vi "Translator.vi"(0 "Input":variant, 11 "error in (no error)":errorcluster) -> (4 "Output":variant, 15 "error out":errorcluster)   [LabVIEW 2014, in "Arduino LiquidCrystal Wrapper.lvlib"]
doc: "An example of how to create the Translator to convert the LabVIEW VIs to Arduino C code."
uses:
  <vilib>/Aledyne-TSXperts/Arduino Compatible Compiler for LabVIEW/addons/Arduino LiquidCrystal Wrapper/Arduino LiquidCrystal Wrapper.lvlib
panel:
  out "Outputs":string[](array[string])
  out "Inputs":string[](array[string])
  out "Output Datatypes":string[](array[string])
  out "Input Datatypes":string[](array[string])
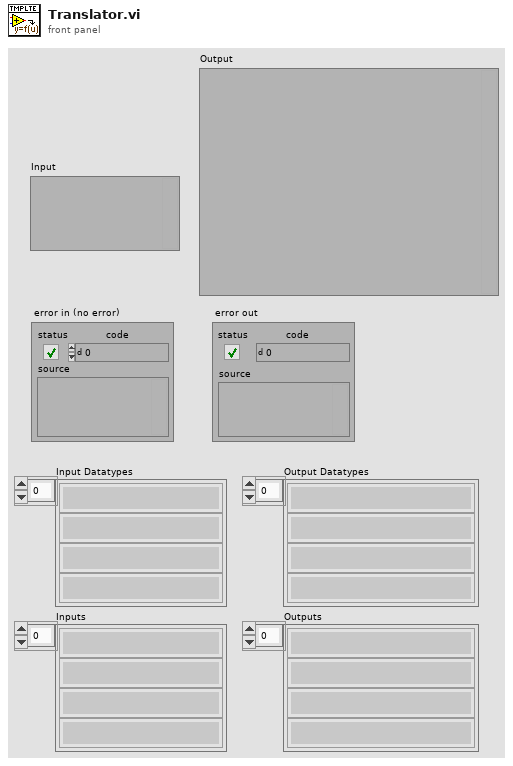
[diagram p1: front panel]
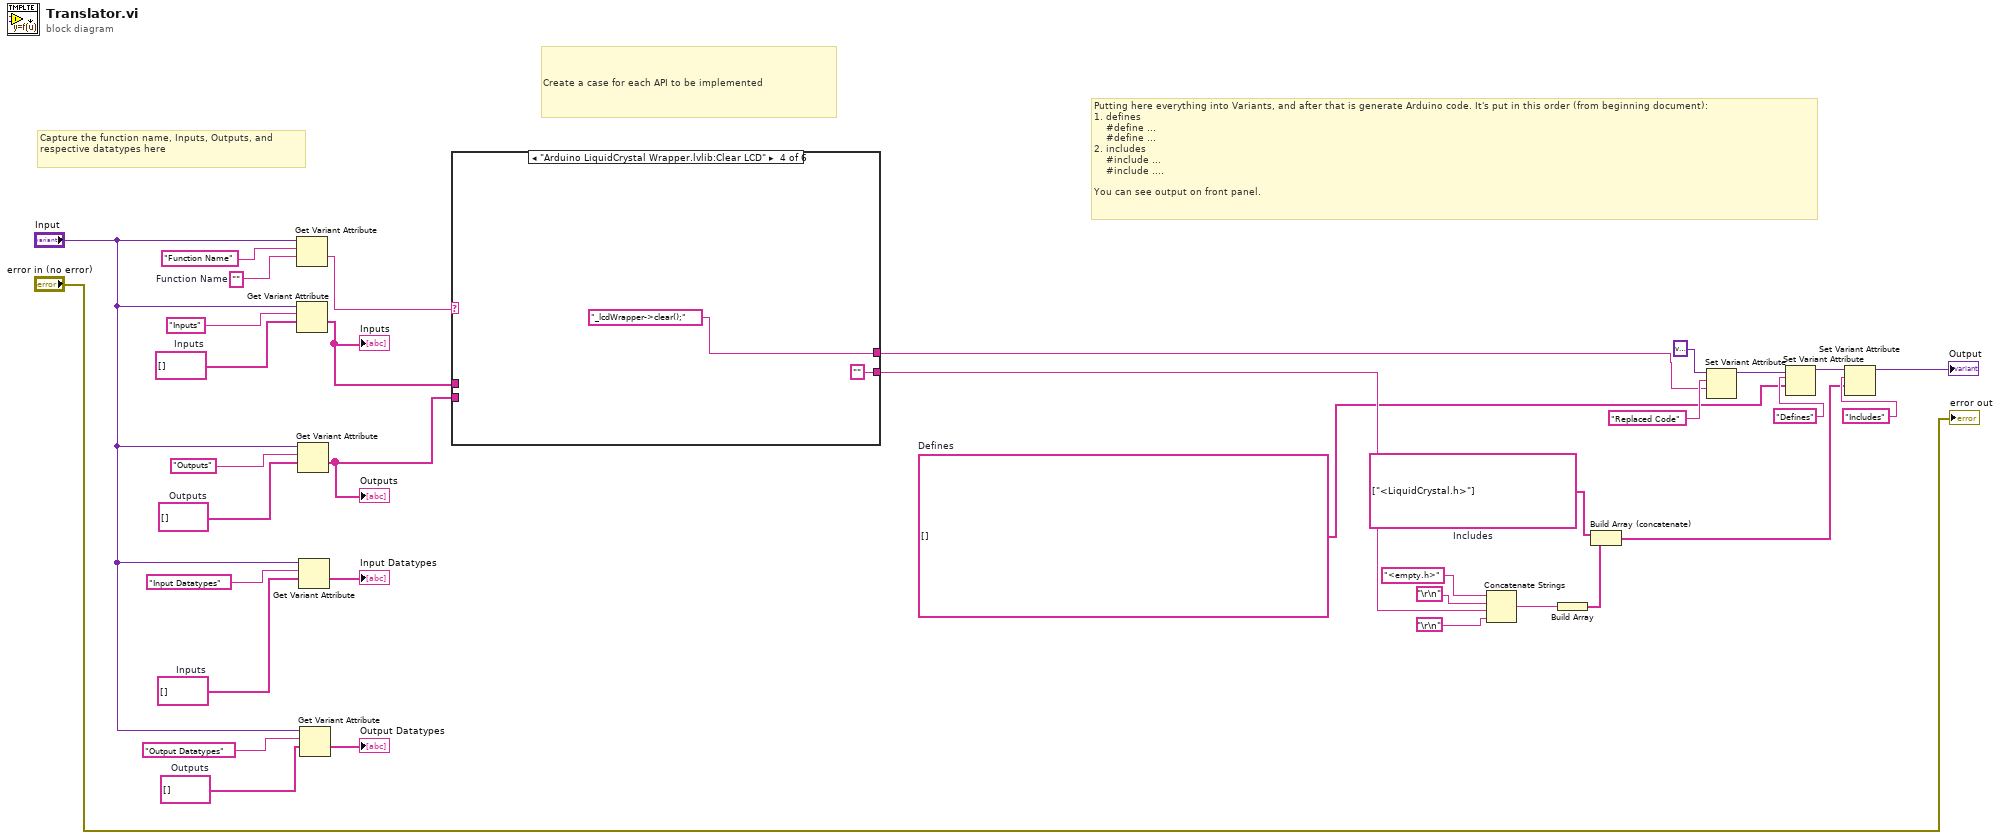
[diagram p0: block diagram]
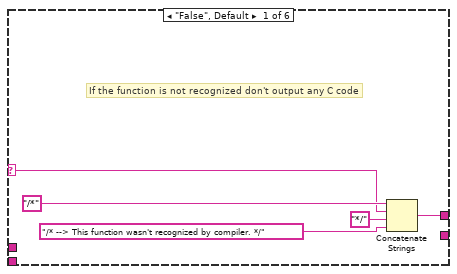
[diagram p2: hidden frame]
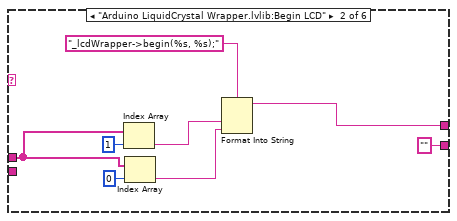
[diagram p3: hidden frame]
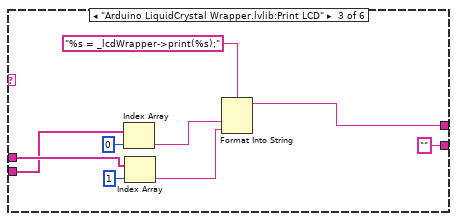
[diagram p4: hidden frame]
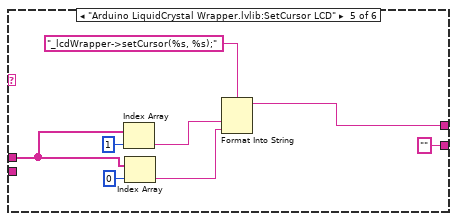
[diagram p5: hidden frame]
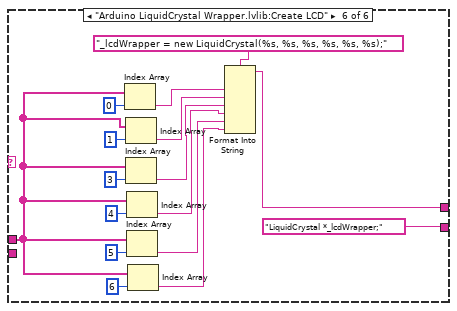
[diagram p6: hidden frame]
diagram:
  w1 = string[] []  # Defines
  w21 = string[] []  # Outputs
  w22 = string[] []  # Inputs
  w3 = string[] ["<LiquidCrystal.h>"]  # Includes
  w30 = string[] []  # Outputs
  w31 = string[] []  # Inputs
  w32 = ""  # Function Name
  # "Capture the function name, Inputs, Outputs, and respective datatypes here"
  # "Putting here everything into Variants, and after that is generate Arduino code. It's put in this order (from beginning document):\n1. defines\n    #define ...\n    #define ...\n2. includes\n    #include ...\n    #include ....\n\nYou can see output on front panel."
  # "Create a case for each API to be implemented"
  n1 = Get Variant Attribute(Variant="Input", name="Function Name", default value (empty Variant)=w32) -> (value=w27:string)  [unwired: 1 in, 3 out]
  n2 = Get Variant Attribute(Variant="Input", name="Inputs", default value (empty Variant)=w31) -> (value=w17:string[])  [unwired: 1 in, 3 out]
  "Inputs" <- w17
  n3 = Get Variant Attribute(Variant="Input", name="Outputs", default value (empty Variant)=w30) -> (value=w18:string[])  [unwired: 1 in, 3 out]
  "Outputs" <- w18
  n4 = Get Variant Attribute(Variant="Input", name="Input Datatypes", default value (empty Variant)=w22) -> (value=→"Input Datatypes":string[])  [unwired: 1 in, 3 out]
  n5 = Get Variant Attribute(Variant="Input", name="Output Datatypes", default value (empty Variant)=w21) -> (value=→"Output Datatypes":string[])  [unwired: 1 in, 3 out]
  n6 = case shown="\"Arduino LiquidCrystal Wrapper.lvlib:Clear LCD\"" w27 {
    selector: w27 -> [w37 _ _ _ _ _]
    tunnel: [w35 w41 w50 "_lcdWrapper->clear();" w61 w68] -> w26
    tunnel: w17 -> [_ w46 w55 _ w59 w72]
    tunnel: w18 -> [_ _ w48 _ _ _]
    tunnel: [_ "" "" "" "" "LiquidCrystal *_lcdWrapper;"] -> w9
    frame "False", Default {
      # "If the function is not recognized don't output any C code"
      n7 = Concatenate Strings("/*" ("name"), w37, "*/" ("name"), "/* --> This function wasn't recognized by compiler. */" ("name")) -> (w35:string)
    }
    frame "Arduino LiquidCrystal Wrapper.lvlib:Begin LCD" {
      n8 = Index Array(array=w46, index=1) -> (element=w42:string)
      n9 = Index Array(array=w46, index=0) -> (element=w43:string)
      n10 = Format Into String(format string="_lcdWrapper->begin(%s, %s);", w42, w43) -> (resulting string=w41:string)  [unwired: 2 in, 1 out]
    }
    frame "Arduino LiquidCrystal Wrapper.lvlib:Print LCD" {
      n11 = Index Array(array=w48, index=0) -> (element=w51:string)
      n12 = Index Array(array=w55, index=1) -> (element=w52:string)
      n13 = Format Into String(format string="%s = _lcdWrapper->print(%s);", w51, w52) -> (resulting string=w50:string)  [unwired: 2 in, 1 out]
    }
    frame "Arduino LiquidCrystal Wrapper.lvlib:Clear LCD" {
    }
    frame "Arduino LiquidCrystal Wrapper.lvlib:SetCursor LCD" {
      n14 = Index Array(array=w59, index=1) -> (element=w62:string)
      n15 = Index Array(array=w59, index=0) -> (element=w63:string)
      n16 = Format Into String(format string="_lcdWrapper->setCursor(%s, %s);", w62, w63) -> (resulting string=w61:string)  [unwired: 2 in, 1 out]
    }
    frame "Arduino LiquidCrystal Wrapper.lvlib:Create LCD" {
      n17 = Index Array(array=w72, index=0) -> (element=w79:string)
      n18 = Index Array(array=w72, index=1) -> (element=w80:string)
      n19 = Index Array(array=w72, index=3) -> (element=w73:string)
      n20 = Index Array(array=w72, index=4) -> (element=w71:string)
      n21 = Index Array(array=w72, index=5) -> (element=w70:string)
      n22 = Index Array(array=w72, index=6) -> (element=w69:string)
      n23 = Format Into String(format string="_lcdWrapper = new LiquidCrystal(%s, %s, %s, %s, %s, %s);", w79, w80, w73, w71, w70, w69) -> (resulting string=w68:string)  [unwired: 2 in, 1 out]
    }
  }
  n24 = Concatenate Strings("<empty.h>" ("string"), "\r\n", w9, "\r\n") -> (w12:string)
  n25 = Build Array(w12) -> (w2:string[])
  n26 = Build Array (concatenate)(w3, w2) -> (w4:string[])
  n27 = Set Variant Attribute(Variant=variant ("variant"), name="Replaced Code", value=w26) -> (Variant out=w7:variant)  [unwired: 1 in, 2 out]
  n28 = Set Variant Attribute(Variant=w7, name="Defines", value=w1) -> (Variant out=w6:variant)  [unwired: 1 in, 2 out]
  n29 = Set Variant Attribute(Variant=w6, name="Includes", value=w4) -> (Variant out=→"Output":variant)  [unwired: 1 in, 2 out]
  "error out" <- "error in (no error)"
